vi "Camera.SetData.vi"(8 "error in (no error)":errorcluster, 10 "Value":T1, 11 "Camera":refnum<class "Camera.lvclass">) -> (0 "error out":errorcluster, 3 "Camera out":refnum<class "Camera.lvclass">)   [LabVIEW 2015]
doc: "---------------------------------------------------------------\nJKI State Machine Objects™\nhttp://jki.net/state-machine-objects/\nCopyright (C) 2005-2015, JKI <info@jki.net>\nALL RIGHTS RESERVEDJKI State Machine Objects (SMO) 1.0.0.5\nJKI - JKI\nCopyright (c) 2016, JKI"
uses:
  Typedefs/ValueChanged--EventData--Cluster.ctl
  Camera.lvclass
  Typedefs/Value.ctl
panel:
  # "For instructions on how to use the JKI State Machine Objects, examples and video tutorials, visit:\nhttp://jki.net/state-machine-objects/\n\nJKI State Machine Objects™\nhttp://jki.net/state-machine-objects/\nCopyright (C) 2005-2015, JKI <info@jki.net>\nALL RIGHTS RESERVED"
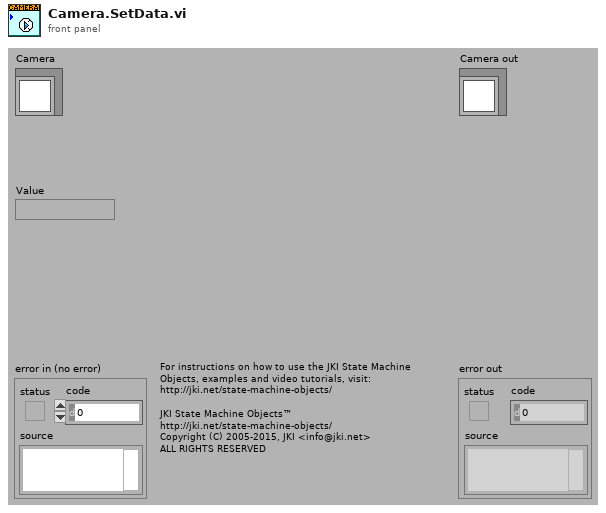
[diagram p1: front panel]
types:
  T1 = typedef "Value.ctl" = string
  T2 = typedef "ValueChanged--EventData--Cluster.ctl" = cluster{"New Value":string}
  T3 = typedef "Camera.lvclass/PrivateData--Ref.ctl" = refnum<data-value>
  T4 = typedef "Camera.lvclass/PrivateData--Cluster.ctl" = cluster{"Public Events":T5, "Protected Events":T6, "Private Events":T7, "Dependencies":T8}
  T5 = typedef "Camera.lvclass/PublicEvents--Cluster.ctl" = cluster{"NewImage":refnum<user-event>, "ImageSaved":refnum<user-event>}
  T6 = typedef "Camera.lvclass/ProtectedEvents--Cluster.ctl" = cluster{"placeholder":refnum<user-event>}
  T7 = typedef "Camera.lvclass/PrivateEvents--Cluster.ctl" = cluster{"New Value":refnum<user-event>, "Grab Image":refnum<user-event>, "Save Image":refnum<user-event>, "Get Image":refnum<user-event>}
  T8 = typedef "Camera.Simulated.lvclass/Dependencies--Cluster.ctl" = cluster{"CircularBuffer.ImageData":refnum<class "CircularBuffer.ImageData.lvclass">}
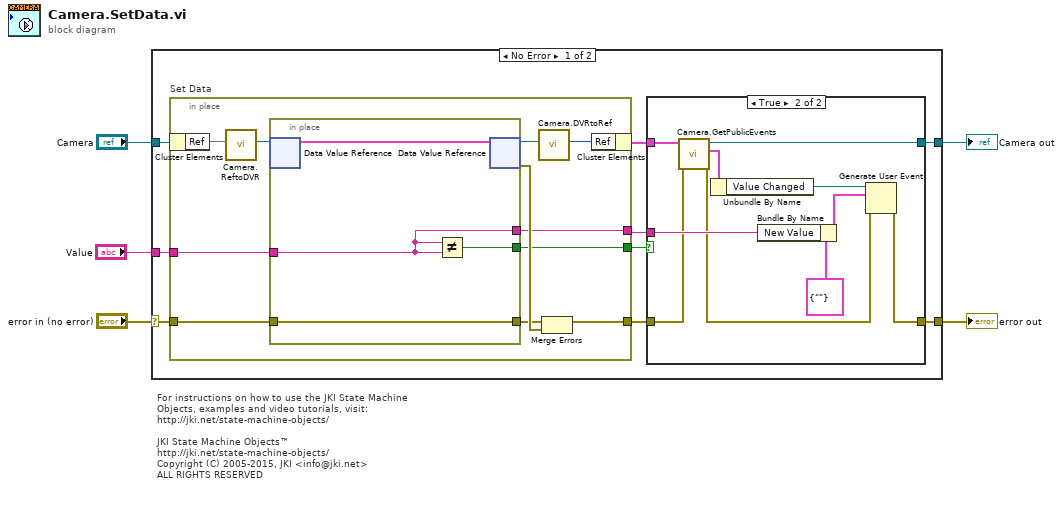
[diagram p0: block diagram]
diagram:
  # "For instructions on how to use the JKI State Machine Objects, examples and video tutorials, visit:\nhttp://jki.net/state-machine-objects/\n\nJKI State Machine Objects™\nhttp://jki.net/state-machine-objects/\nCopyright (C) 2005-2015, JKI <info@jki.net>\nALL RIGHTS RESERVED"
  n1 = case shown="No Error" "error in (no error)" {
    selector: "error in (no error)" -> [w12 w42]
    tunnel: "Camera" -> [w13 w43]
    tunnel: [w10 w42] -> w4
    tunnel: [w8 w43] -> w3
    tunnel: "Value" -> [w14 _]
    frame No Error {
      n2 = in-place "Set Data" {
        in-place-border: w12 -> [w37]
        in-place-border: [w34] -> w7
        in-place-border: w14 -> [w33]
        in-place-border: [w32] -> w11
        in-place-border: [w27] -> w6
        n3 = in-place-cluster #1(w13) -> ("Ref"=w31)
        n4 = call "Camera.ReftoDVR.vi"("Ref"=w31) -> ("Ref"=w30:T3)  [unwired: 10 in]
        n5 = in-place {
          in-place-border: w37 -> [w41]
          in-place-border: [w41] -> w35
          in-place-border: w33 -> [w39]
          in-place-border: [w39] -> w32
          in-place-border: [w40] -> w27
          n6 = in-place-dvr #2(w30) -> (w38:T4)  [unwired: 1 out]
          n7 = Not Equal?(x=w39, y=w39) -> (x != y?=w40:bool)
          n8 = in-place-dvr #2(w38) -> (w29:T3, w36:errorcluster)
        }
        n9 = call "Camera.DVRtoRef.vi"("Ref"=w29) -> ("Ref"=w28:u32)  [unwired: 10 in]
        n10 = Merge Errors(w35, w36) -> (w34:errorcluster)
        n11 = in-place-cluster #1("Ref"=w28) -> (w9:cluster{})
      }
      n12 = case shown="True" w6 {
        tunnel: w11 -> [_ w23]
        tunnel: [w15 w22] -> w10
        tunnel: w9 -> [w16 w21]
        tunnel: [w16 w20] -> w8
        tunnel: w7 -> [w15 w18]
        frame False {
        }
        frame True {
          n13 = call "Camera.GetPublicEvents.vi"("error in (no error)"=w18, "Camera"=w21) -> ("error out"=w17:errorcluster, "Camera Public Events"=w19:T5, "Camera out"=w20:refnum<class "Camera.lvclass">)  [unwired: 7 in]
          n14 = Unbundle By Name(w19) -> ("Value Changed"=w26:refnum<user-event>)
          n15 = Bundle By Name(cluster=T2 {"New Value"=""} ("event data"), "New Value"=w23) -> (w24:T2)
          n16 = Generate User Event(user event=w26, event data cluster=w24, error in=w17) -> (error out=w22:errorcluster)  [unwired: 1 in, 1 out]
        }
      }
    }
    frame Error {
    }
  }
  "error out" <- w4
  "Camera out" <- w3
